vi "VI Tree.vi"   [LabVIEW 2023, in "Error Manager.lvlib" / "Error Log.lvclass"]
uses:
  Error Log.lvclass
  Error Log.lvclass/Error Log.ctl
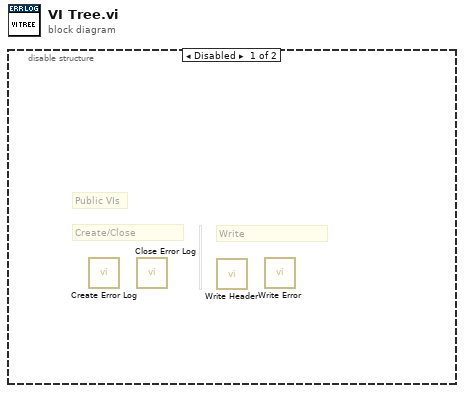
[diagram p0: block diagram]
diagram:
  n1 = disable-structure shown="Disabled" {
    frame Disabled {
      # "Write"
      # "Create/Close"
      # "Public VIs"
      n2 = call "Create Error Log.vi"() -> ()  [unwired: 9 in, 3 out]
      n3 = call "Close Error Log.vi"() -> ()  [unwired: 11 in, 1 out]
      n4 = call "Write Header.vi"() -> ()  [unwired: 11 in, 1 out]
      n5 = call "Write Error.vi"() -> ()  [unwired: 11 in, 1 out]
    }
    frame Enabled {
    }
  }
